vi "Konfig Dateien laden-speichern.vi"(6 "Aktion":T1=enum."laden", 8 "Fehler (Eingang)":errorcluster, 11 "Software Version":string) -> (0 "Fehler (Ausgang)":errorcluster)   [LabVIEW 2020, in "Konfig-Dateien.lvlib"]
uses:
  Konfig-Dateien.lvlib
  Aktionen Konfig.ctl
  Betriebsstundenzaehler/FGV BSZ Aktionen.ctl
  Stickstoff Befuellung/Aktionen Stockstoff Befuellung.ctl
  FGV Betriebsdaten Aktionen.ctl
  Allgemein/FGV Zustaende Aktionen.ctl
  SysLog/SysLog Interface cRIO.ctl
  Externe Stickstoff Befuellung/Aktionen Externe Stockstoff Befuellung.ctl
  CAN Interface/FGV CAN Daten Aktionen.ctl
  <vilib>/Utility/config.llb/Write Key (U32).vi
  <vilib>/Utility/config.llb/Write Key (String).vi
  Betriebsstundenzaehler/Betriebsstundenzaehler.lvlib
  Stickstoff Befuellung/Stickstoff Befuellung.lvlib
  Allgemein/Allgemein.lvlib
  SysLog/SysLog_cRIO.lvlib
  <vilib>/Utility/config.llb/NI_LVConfig.lvlib
  Externe Stickstoff Befuellung/Externe Stickstoff Befuellung.lvlib
  CAN Interface/CAN Interface.lvlib
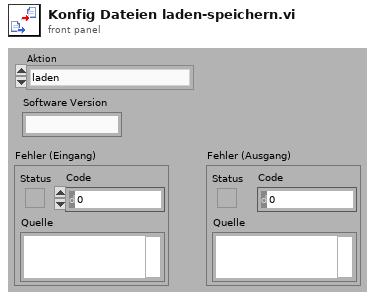
[diagram p1: front panel]
types:
  T1 = typedef "Konfig-Dateien.lvlib/Aktionen Konfig.ctl" = enum16{"lesen", "laden", "speichern  System.ini", "speichern Anlagengrenzw.", "speichern PID + Sonstige", "speichern BSZ BMP", "speichern BSZ FT-IR", "speichern Stickstoff Bef.", "speichern Ext. Stickstoff Bef.", "speichern CAN_Konfig"}
  T2 = typedef "Allgemein.lvlib/FGV Zustaende Aktionen.ctl" = enum16{"lesen", "Zustand PC", "Zustand cRIO", "Bildnummer", "Samplepoint", "Sysloglevel"}
  T3 = typedef "Konfig-Dateien.lvlib/FGV Betriebsdaten Aktionen.ctl" = enum16{"lesen", "Anlagengrenzw.", "PID Param.", "Sonstige", "Sensor Para."}
  T4 = typedef "Stickstoff Befuellung.lvlib/Aktionen Stockstoff Befuellung.ctl" = enum16{"lesen", "Befüllen vorbereiten", "Befüllen", "Befüllen beenden", "Warten", "deaktiviert", "initialisieren", "anstehender Fehler"}
  T5 = typedef "Betriebsstundenzaehler.lvlib/FGV BSZ Aktionen.ctl" = enum16{"Lesen", "Initialisieren", "Starten Pumpe", "Zählen Pumpe", "Starten FT-IR", "Zählen FT-IR"}
  T6 = typedef "CAN Interface.lvlib/FGV CAN Daten Aktionen.ctl" = enum16{"lesen", "Daten", "Konfig", "laden", "speichern", "Status"}
  T7 = typedef "Externe Stickstoff Befuellung.lvlib/Aktionen Externe Stockstoff Befuellung.ctl" = enum16{"lesen", "Befüllen vorbereiten", "Befüllen", "Befüllen beenden", "Warten", "deaktiviert", "initialisieren"}
  T8 = typedef "SysLog_cRIO.lvlib/SysLog Interface cRIO.ctl" = cluster{"FehlermeldungsCode":i32, "ErfolgsmeldungsCode":i32, "ParameterListenString":string, "intern":bool}
  T9 = typedef "Anlagengrenzwerte.lvlib/Anlagen-Grenzwerte Anzeige.ctl" = cluster{"Eingangsdruck FT-IR:":T10, "Durchfluss FT-IR:":T10, "Durchfluss CalGas:":T10, "Druck Ausgang:":T10, "Druck Kalter Block:":T10, "Heizleitungen intern:":T10, "Heizleitung zu FT-IR:":T10, "Heizung Filterblock:":T10, "Heizung Pumpe:":T10, "Heizleitung Extern SP1:":T10, "Heizleitung Extern SP2:":T10, "FT-IR Heizung Messzelle:":T10, "Schaltschranktemperatur:":T10, "Gaskühler:":T10}
  T10 = typedef "Anlagengrenzwerte.lvlib/Anlagen-Parameter Anzeige.ctl" = cluster{"Sollwert":sgl, "Warn-Min":sgl, "Warn-Max":sgl, "Abschalt-Min":sgl, "Abschalt-Max":sgl, "Regler":u16}
  T11 = typedef "Erweiterte Konfig.lvlib/PID-Parameter Anzeige.ctl" = cluster{"Heizung\nFilterblock":T12, "Heizung\nPumpe":T12, "Heizung\nHeizleitungen":T12, "Heizleitung\nExtern":T12, "Heizung\nFB-Druckregler":T12}
  T12 = typedef "Erweiterte Konfig.lvlib/PID-Parameter.ctl" = cluster{"P-Anteil":T13, "I-Anteil":T13, "D-Anteil":T13, "Regelzonengr.":T13, "max. OUT":T13}
  T13 = typedef "Zahlen-Eingabefeld.ctl" = sgl
  T14 = typedef "Erweiterte Konfig.lvlib/Sonstige Parameter.ctl" = cluster{"Lüfter langsam":sgl, "Lüfter schnell":sgl, "FT-IR Kühlung Soll":sgl, "FT-IR Kühlung Max":sgl, "Überwachung":T15, "Befüllung aktiv":T16, "Stickstoff Befüllzeit":sgl, "Befüllintervall":sgl, "Kalibrierwert FT-IR":sgl, "Offset Ausgang":sgl, "Offset FT-IR":sgl, "Offset Druck FT-IR":sgl, "Dichtheitstest Zeit":sgl, "Dichtheitstest Abfall":sgl, "Dichtheitstest Umfang":T17, "Offset Umgebung":sgl, "Max Taupunkt":sgl, "Pumpendrehzahl":sgl, "ext. Befüllung":T16, "Ext. Stickstoff Befüllzeit":sgl}
  T15 = typedef "Auswahlfeld.ctl" = u16
  T16 = typedef "LogKonfig.lvlib/Auswahlfeld aktiviert-deaktiviert.ctl" = u16
  T17 = typedef "Erweiterte Konfig.lvlib/Dichtheitstest Umfang.ctl" = u16
  T18 = cluster{"PID-Parameter Anzeige":T11, "Sonstige":T14, "Parameter Sensoren":cluster{"Kal.Durchfl.FTIR":sgl, "Kal.Durchfl.PMA":sgl, "Offset Durchfl.FTIR":sgl, "Offset Druck Ausgang":sgl, "Offset Druck Umgebung":sgl, "Offset Durchfl.PMA":sgl, "Offset Druck CG PMA":sgl, "Offset Druck CG":sgl, "Offset Druck FTIR IAG":sgl, "Druck Kalter Block":sgl}}
  T19 = typedef "Stickstoff Befuellung.lvlib/Stickstoff Befuellzeiten.ctl" = cluster{"Zeitstempel 1":timestamp, "Zeitstempel 2":timestamp, "Befülldauer":sgl}
  T20 = typedef "CAN Konfig.lvlib/Konfig Daten PC.ctl" = cluster{"Baude Rate":T21, "COM state":u8, "Frame-ID FTIR Start":u32, "Frame-ID FTIR End":u32, "Frame-ID Status Start":u32, "Frame-ID Status End":u32, "Zustand Information":u32, "Aktion":u32, "Frame-ID FTIR Arry":u32[], "Frame-ID Status Arry":u32[], "GPS Start":u32, "Interface":refnum<k21>}
  T21 = typedef "CAN Interface.lvlib/Baude Rate.ctl" = u32
  T22 = cluster{"Kal.Durchfl.FTIR":sgl, "Kal.Durchfl.PMA":sgl, "Offset Durchfl.FTIR":sgl, "Offset Druck Ausgang":sgl, "Offset Druck Umgebung":sgl, "Offset Durchfl.PMA":sgl, "Offset Druck CG PMA":sgl, "Offset Druck CG":sgl, "Offset Druck FTIR IAG":sgl, "Druck Kalter Block":sgl}
  T23 = cluster{"SysLogLevel":u16, "Software Version":string}
  T24 = cluster{"Lüfter langsam":sgl, "Lüfter schnell":sgl, "FT-IR Kühlung Soll":sgl, "FT-IR Kühlung Max":sgl, sgl, sgl, "Stickstoff Befüllzeit":sgl, "Befüllintervall":sgl, "Kalibrierwert FT-IR":sgl, "Offset Ausgang":sgl, "Offset FT-IR":sgl, "Offset Druck FT-IR":sgl, "Dichtheitstest Zeit":sgl, "Dichtheitstest Abfall":sgl, sgl, "Offset Umgebung":sgl, "Max Taupunkt":sgl, "Pumpendrehzahl":sgl, sgl, "Ext. Stickstoff Befüllzeit":sgl}
  T25 = cluster{"Sollwert":sgl, "Warn-Min":sgl, "Warn-Max":sgl, "Abschalt-Min":sgl, "Abschalt-Max":sgl, "Regler":sgl}
  T26 = typedef "NI_LVConfig.lvlib/Config Data RefNum.ctl" = refnum<k1>
  T27 = typedef "Erweiterte Konfig.lvlib/Parameter Sensoren.ctl" = cluster{"Kal.Durchfl.FTIR":sgl, "Kal.Durchfl.PMA":sgl, "Offset Durchfl.FTIR":sgl, "Offset Druck Ausgang":sgl, "Offset Druck Umgebung":sgl, "Offset Durchfl.PMA":sgl, "Offset Druck CG PMA":sgl, "Offset Druck CG":sgl, "Offset Druck FTIR IAG":sgl, "Druck Kalter Block":sgl}
  T28 = cluster{"PID-Parameter":T11, "Sonstige":T14, "Parameter Sensoren":T27}
  T29 = cluster{"Befüllen 1":timestamp, "Befüllen 2":timestamp, "Befülldauer":sgl}
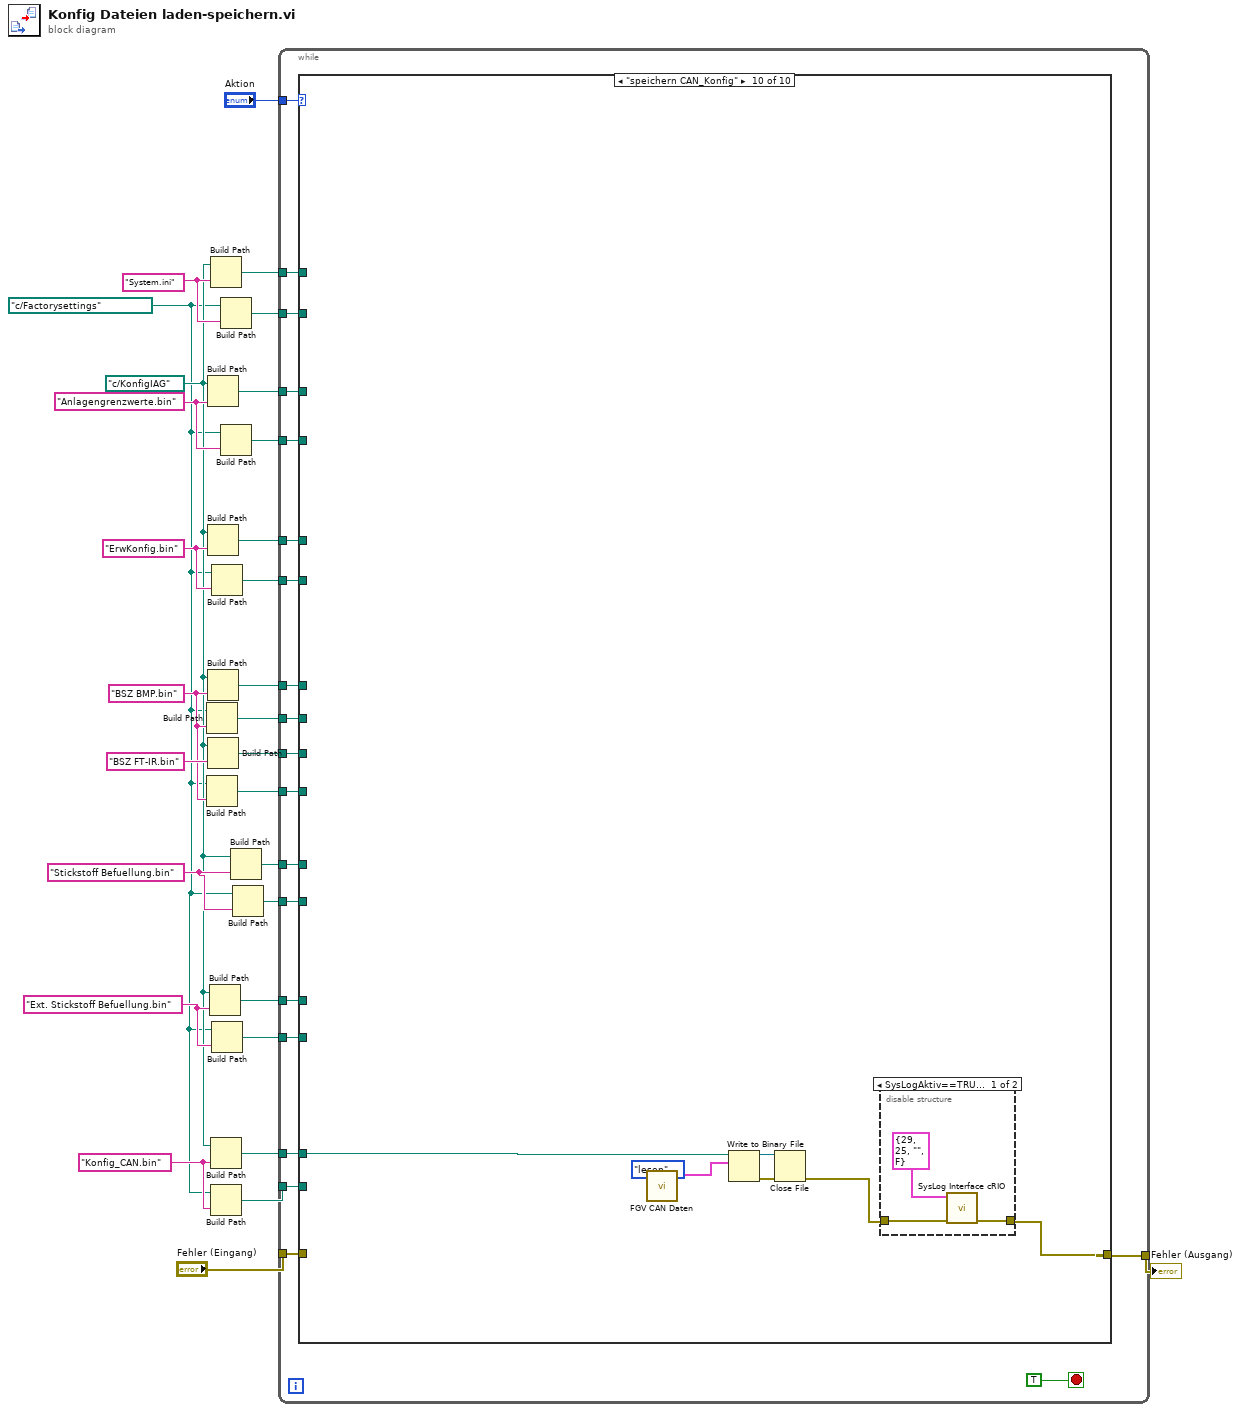
[diagram p0: block diagram]
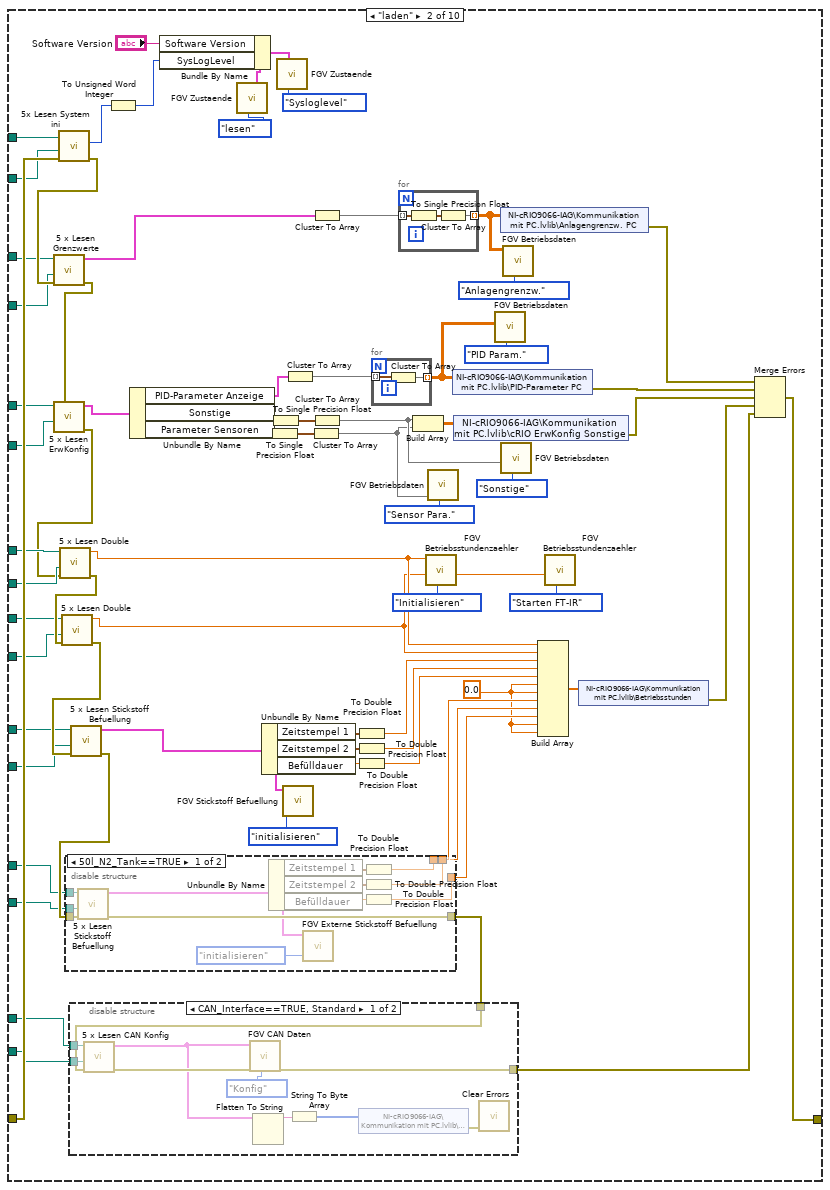
[diagram p3: hidden frame]
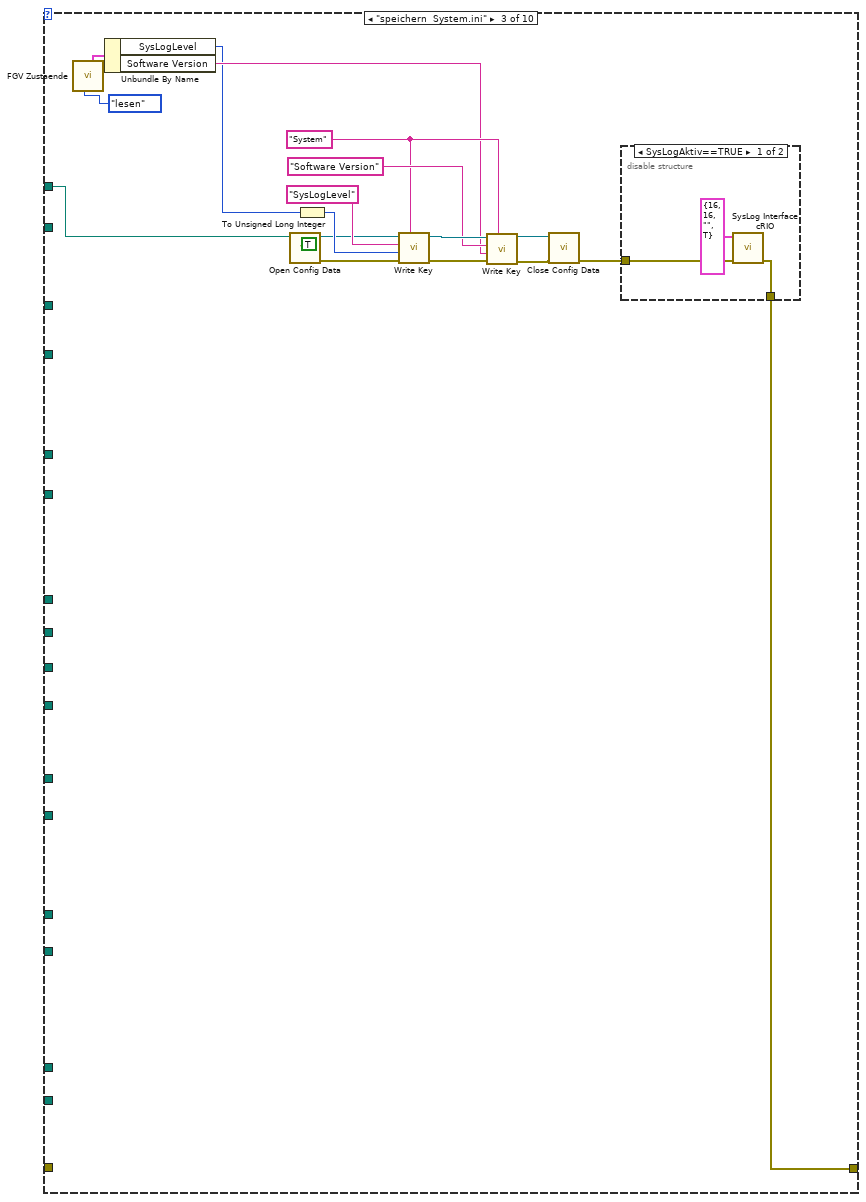
[diagram p6: hidden frame]
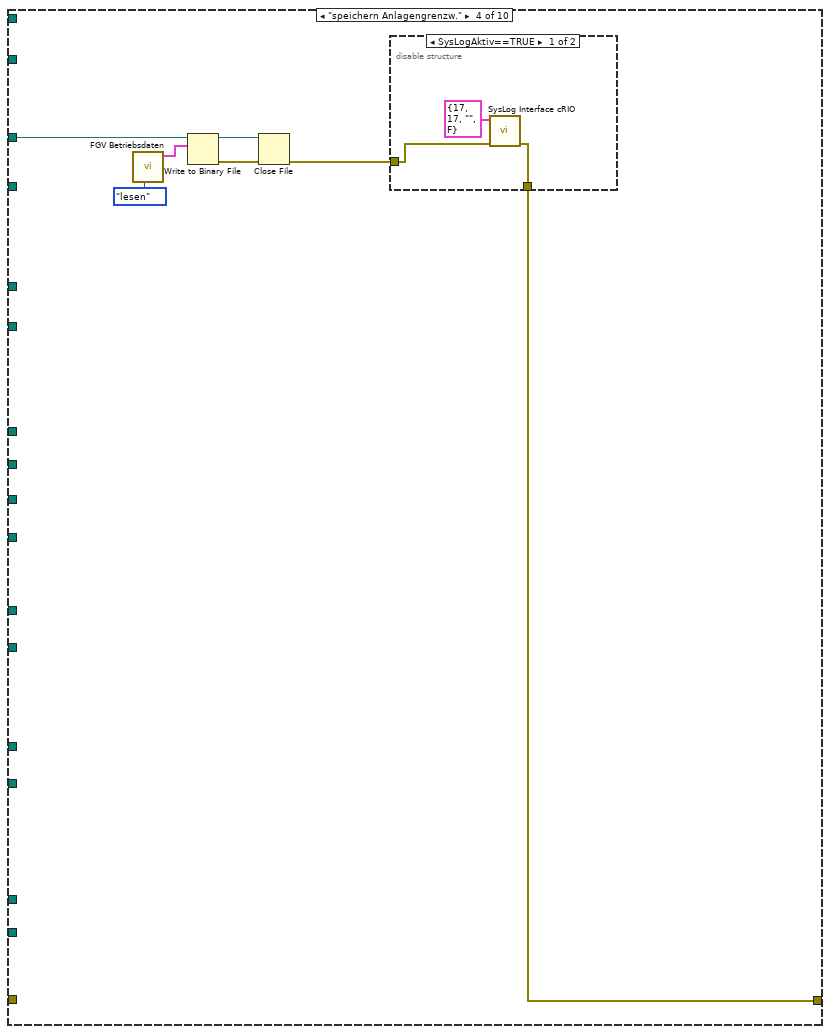
[diagram p8: hidden frame]
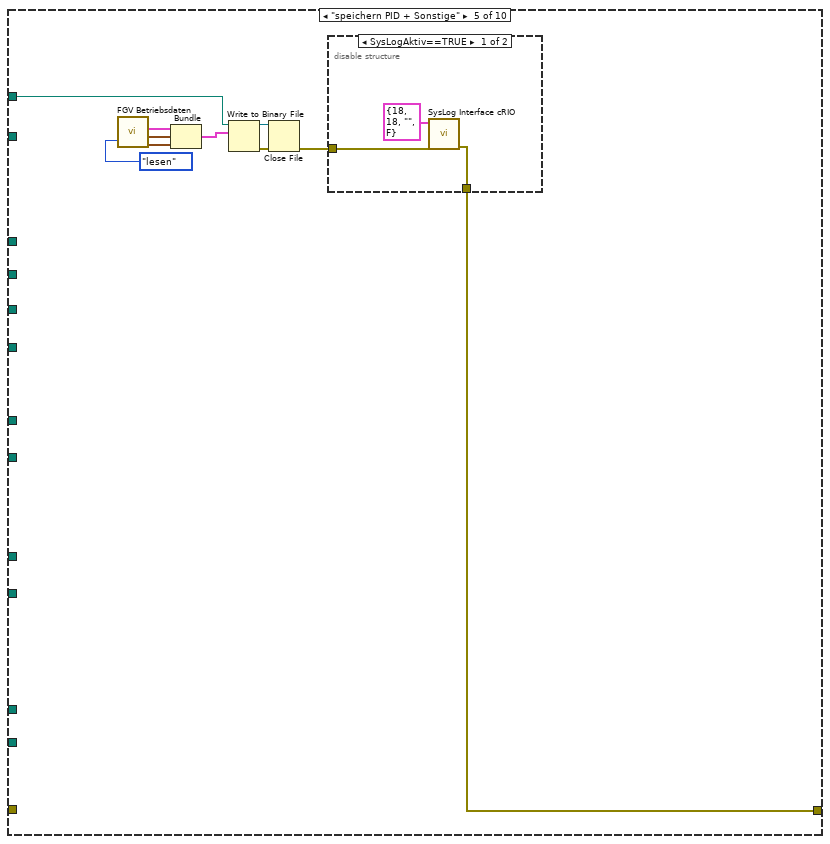
[diagram p10: hidden frame]
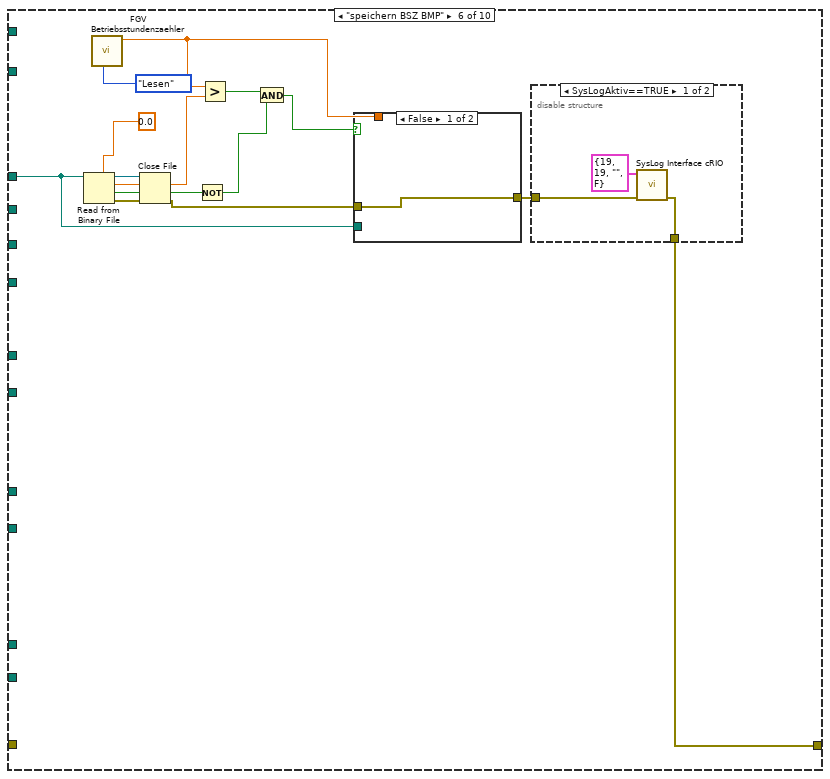
[diagram p12: hidden frame]
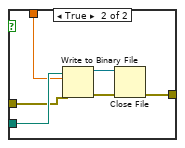
[diagram p14: hidden frame]
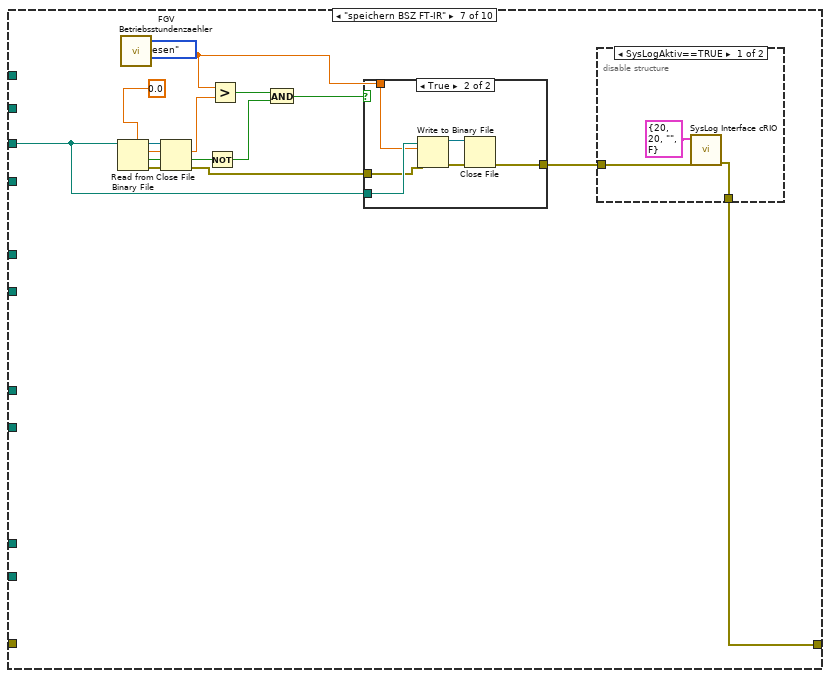
[diagram p15: hidden frame]
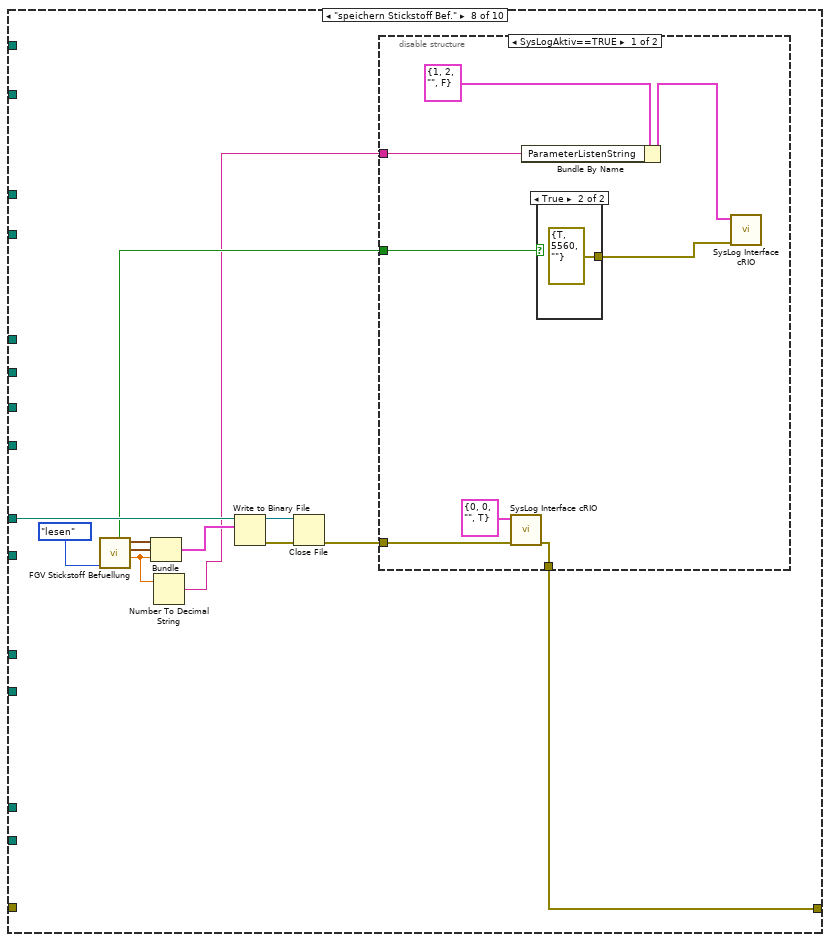
[diagram p18: hidden frame]
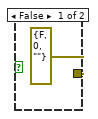
[diagram p19: hidden frame]
diagram:
  w5 = "Konfig_CAN.bin" ("Dateiname")
  w8 = "Ext. Stickstoff Befuellung.bin" ("Dateiname")
  w3 = path "c:/Factorysettings" ("Applikation:Verzeichnispfad")
  w21 = "System.ini" ("Name oder relativer Pfad")
  w13 = "Stickstoff Befuellung.bin" ("Dateiname")
  w15 = "BSZ BMP.bin" ("Dateiname")
  w16 = "ErwKonfig.bin" ("Name oder relativer Pfad")
  w4 = path "c:/KonfigIAG" ("Applikation:Verzeichnispfad")
  w19 = "Anlagengrenzwerte.bin" ("Name oder relativer Pfad")
  n1 = Build Path(base path=w3, name or relative path=w15) -> (appended path=w9:path)
  n2 = Build Path(base path=w3, name or relative path=w15) -> (appended path=w11:path)
  n3 = Build Path(base path=w4, name or relative path=w19) -> (appended path=w28:path)
  n4 = Build Path(base path=w4, name or relative path=w16) -> (appended path=w17:path)
  n5 = Build Path(base path=w4, name or relative path=w15) -> (appended path=w27:path)
  n6 = Build Path(base path=w4, name or relative path="BSZ FT-IR.bin" ("Dateiname")) -> (appended path=w25:path)
  n7 = Build Path(base path=w4, name or relative path=w8) -> (appended path=w7:path)
  n8 = Build Path(base path=w4, name or relative path=w21) -> (appended path=w24:path)
  n9 = Build Path(base path=w4, name or relative path=w5) -> (appended path=w2:path)
  n10 = Build Path(base path=w3, name or relative path=w5) -> (appended path=w1:path)
  n11 = Build Path(base path=w3, name or relative path=w16) -> (appended path=w10:path)
  n12 = Build Path(base path=w3, name or relative path=w8) -> (appended path=w6:path)
  n13 = Build Path(base path=w3, name or relative path=w21) -> (appended path=w20:path)
  n14 = Build Path(base path=w3, name or relative path=w19) -> (appended path=w18:path)
  n15 = Build Path(base path=w4, name or relative path=w13) -> (appended path=w14:path)
  n16 = Build Path(base path=w3, name or relative path=w13) -> (appended path=w12:path)
  n17 = while {
    tunnel: "Aktion" -> [w46]
    tunnel: w17 -> [w47]
    tunnel: w28 -> [w48]
    tunnel: w27 -> [w45]
    tunnel: w25 -> [w44]
    tunnel: w14 -> [w43]
    tunnel: w24 -> [w42]
    tunnel: [w41] -> w23
    tunnel: "Fehler (Eingang)" -> [w40]
    tunnel: w20 -> [w39]
    tunnel: w18 -> [w38]
    tunnel: w12 -> [w37]
    tunnel: w11 -> [w36]
    tunnel: w10 -> [w35]
    tunnel: w9 -> [w34]
    tunnel: w7 -> [w33]
    tunnel: w6 -> [w32]
    tunnel: w2 -> [w31]
    tunnel: w1 -> [w30]
    stop <- TRUE stop-if-true
    n18 = case shown="\"speichern CAN_Konfig\"" w46 {
      tunnel: w48 -> [_ w79 _ w178 _ _ _ _ _ _]
      tunnel: w47 -> [_ w76 _ _ w191 _ _ _ _ _]
      tunnel: w45 -> [_ w73 _ _ _ w204 _ _ _ _]
      tunnel: w44 -> [_ w68 _ _ _ _ w226 _ _ _]
      tunnel: w43 -> [_ w64 _ _ _ _ _ w254 _ _]
      tunnel: w42 -> [_ w92 w153 _ _ _ _ _ _ _]
      tunnel: [w50 w84 w151 w175 w185 w198 w222 w249 w275 w287] -> w41
      tunnel: w40 -> [w50 w83 _ _ _ _ _ _ _ _]
      tunnel: w39 -> [_ w78 _ _ _ _ _ _ _ _]
      tunnel: w38 -> [_ w80 _ _ _ _ _ _ _ _]
      tunnel: w37 -> [_ w63 _ _ _ _ _ _ _ _]
      tunnel: w36 -> [_ w67 _ _ _ _ _ _ _ _]
      tunnel: w35 -> [_ w75 _ _ _ _ _ _ _ _]
      tunnel: w34 -> [_ w72 _ _ _ _ _ _ _ _]
      tunnel: w33 -> [_ w60 _ _ _ _ _ _ w270 _]
      tunnel: w32 -> [_ w59 _ _ _ _ _ _ _ _]
      tunnel: w31 -> [_ w54 _ _ _ _ _ _ _ w289]
      tunnel: w30 -> [_ w53 _ _ _ _ _ _ _ _]
      frame "lesen", Default {
      }
      frame "laden" {
        w55 = 0.0 ("Element")
        n19 = call "5x Lesen System ini.vi"("Fehler (Eingang, kein Fehler)"=w83, "Factorysettings"=w78, "appended path"=w92) -> ("Fehler (Ausgang)"=w81:errorcluster, "Sys Log Level"=w91:i32)  [unwired: 6 in, 1 out]
        n20 = call "5 x Lesen Grenzwerte.vi"("Fehler (Eingang, kein Fehler)"=w81, "Factorysettings"=w80, "appended path"=w79) -> ("Fehler (Ausgang)"=w77:errorcluster, "Anlagen-Grenzwerte Anzeige"=w82:T9)  [unwired: 6 in, 1 out]
        n21 = call "5 x Lesen ErwKonfig.vi"("Fehler (Eingang, kein Fehler)"=w77, "Factorysettings"=w75, "appended path"=w76) -> ("Fehler (Ausgang)"=w71:errorcluster, "Erw. Konfig"=w74:T18)  [unwired: 6 in, 1 out]
        n22 = call "5 x Lesen Double.vi"("Fehler (Eingang, kein Fehler)"=w71, "Factorysettings"=w72, "appended path"=w73) -> ("Fehler (Ausgang)"=w69:errorcluster, "Double (Ausgang)"=w70:dbl)  [unwired: 6 in, 1 out]
        n23 = call "5 x Lesen Double.vi"("Fehler (Eingang, kein Fehler)"=w69, "Factorysettings"=w67, "appended path"=w68) -> ("Fehler (Ausgang)"=w65:errorcluster, "Double (Ausgang)"=w66:dbl)  [unwired: 6 in, 1 out]
        n24 = call "5 x Lesen Stickstoff Befuellung.vi"("Fehler (Eingang, kein Fehler)"=w65, "Factorysettings"=w63, "appended path"=w64) -> ("Fehler (Ausgang)"=w61:errorcluster, "Stiskstoff Befüllzeiten"=w62:T19)  [unwired: 6 in, 1 out]
        n25 = disable-structure shown="50l_N2_Tank==TRUE" {
          disable-tunnel: w61 -> [w142 _]
          disable-tunnel: [w141 _] -> w52
          disable-tunnel: w60 -> [w138 _]
          disable-tunnel: w59 -> [w137 _]
          disable-tunnel: [w136 _] -> w58
          disable-tunnel: [w135 _] -> w57
          disable-tunnel: [w134 _] -> w56
          frame condition #0 {
            n26 = call "5 x Lesen Stickstoff Befuellung.vi"("Fehler (Eingang, kein Fehler)"=w142, "Factorysettings"=w137, "appended path"=w138) -> ("Fehler (Ausgang)"=w141:errorcluster, "Stiskstoff Befüllzeiten"=w140:T19)  [unwired: 6 in, 1 out]
            n27 = Unbundle By Name(w140) -> ("Zeitstempel 1"=w143:timestamp, "Zeitstempel 2"=w144:timestamp, "Befülldauer"=w145:sgl)
            n28 = call "FGV Externe Stickstoff Befuellung.vi"("Aktion"=Aktionen_Externe_Stockstoff_Befuellung."initialisieren", "Stiskstoff Befüllzeiten"=w140) -> ()  [unwired: 3 in, 7 out]
            n29 = To Double Precision Float(number=w143) -> (double precision float=w136:dbl)
            n30 = To Double Precision Float(number=w144) -> (double precision float=w135:dbl)
            n31 = To Double Precision Float(number=w145) -> (double precision float=w134:dbl)
          }
          frame condition #1 (active) {
          }
        }
        n32 = disable-structure shown="CAN_Interface==TRUE, Standard" {
          disable-tunnel: w54 -> [w131 _]
          disable-tunnel: w53 -> [w130 _]
          disable-tunnel: w52 -> [w129 w133]
          disable-tunnel: [w128 w133] -> w51
          frame condition #0 {
            n33 = call "5 x Lesen CAN Konfig.vi"("Fehler (Eingang, kein Fehler)"=w129, "Factorysettings"=w130, "appended path"=w131) -> ("Fehler (Ausgang)"=w128:errorcluster, "Konfig Daten 2"=w126:T20)  [unwired: 6 in, 1 out]
            n34 = call "FGV CAN Daten.vi"("Aktionen"=FGV_CAN_Daten_Aktionen."Konfig", "Konfig Daten 2"=w126) -> ()  [unwired: 7 in, 3 out]
            n35 = Flatten To String(anything=w126) -> (data string=w127:string)  [unwired: 3 in, 2 out]
            n36 = String To Byte Array(string=w127) -> (unsigned byte array=w125:u8[])
            n37 = shared-variable "NI-cRIO9066-IAG\\Kommunikation mit PC.lvlib\\CAN_Konfig"(w125) -> (error out=w124:errorcluster)  [unwired: 1 in]
            n38 = call <vilib>:"Clear Errors.vi"("error in (no error)"=w124) -> ()  [unwired: 5 in, 2 out]
          }
          frame condition #1 (active) {
          }
        }
        n39 = To Unsigned Word Integer(number=w91) -> (unsigned 16bit integer=w85:u16)
        n40 = Unbundle By Name(w74) -> ("PID-Parameter Anzeige"=w110:T11, "Sonstige"=w108:T14, "Parameter Sensoren"=w97:T22)
        n41 = call "FGV Zustaende.vi"("Aktionen"=FGV_Zustaende_Aktionen."lesen") -> ("SL SV Cluster"=w88:T23)  [unwired: 6 in, 4 out]
        n42 = Bundle By Name(cluster=w88, "Software Version"="Software Version", "SysLogLevel"=w85) -> (w86:T23)
        n43 = Unbundle By Name(w62) -> ("Zeitstempel 1"=w118:timestamp, "Zeitstempel 2"=w117:timestamp, "Befülldauer"=w116:sgl)
        n44 = To Single Precision Float(number=w97) -> (single precision float=w98:T22)
        n45 = To Single Precision Float(number=w108) -> (single precision float=w109:T24)
        n46 = call "FGV Zustaende.vi"("Aktionen"=FGV_Zustaende_Aktionen."Sysloglevel", "SL SV Cluster"=w86) -> ()  [unwired: 5 in, 5 out]
        n47 = call "FGV Stickstoff Befuellung.vi"("Aktion"=Aktionen_Stockstoff_Befuellung."initialisieren", "Stiskstoff Befüllzeiten"=w62) -> ()  [unwired: 3 in, 7 out]
        n48 = Cluster To Array(cluster=w110) -> (array=w111:T12[])
        n49 = Cluster To Array(cluster=w98) -> (array=w93:sgl[])
        n50 = Cluster To Array(cluster=w82) -> (array=w112:T10[])
        n51 = Cluster To Array(cluster=w109) -> (array=w96:sgl[])
        n52 = To Double Precision Float(number=w118) -> (double precision float=w115:dbl)
        n53 = To Double Precision Float(number=w117) -> (double precision float=w114:dbl)
        n54 = To Double Precision Float(number=w116) -> (double precision float=w113:dbl)
        n55 = for {
          tunnel: w111 -> [w147] mode=indexing
          tunnel: [w146] -> w103 mode=indexing
          n56 = Cluster To Array(cluster=w147) -> (array=w146:T13[])
        }
        n57 = for {
          tunnel: w112 -> [w150] mode=indexing
          tunnel: [w148] -> w106 mode=indexing
          n58 = To Single Precision Float(number=w150) -> (single precision float=w149:T25)
          n59 = Cluster To Array(cluster=w149) -> (array=w148:sgl[])
        }
        n60 = Build Array(w96, w93) -> (w94:sgl[][])
        n61 = call "FGV Betriebsstundenzaehler.vi"("BSZ Aktionen"=FGV_BSZ_Aktionen."Initialisieren", "Betriebsstunden FT-IR"=w66, "Betriebsstunden Pumpe"=w70) -> ("Betriebsstunden FT-IR"=w121:dbl)  [unwired: 7 in, 1 out]
        n62 = call "FGV Betriebsdaten.vi"("Aktionen"=FGV_Betriebsdaten_Aktionen."Sensor Para.", "Parameter Sensoren"=w93) -> ()  [unwired: 6 in, 4 out]
        n63 = shared-variable "NI-cRIO9066-IAG\\Kommunikation mit PC.lvlib\\PID-Parameter PC"(w103) -> (error out=w100:errorcluster)  [unwired: 1 in]
        n64 = shared-variable "NI-cRIO9066-IAG\\Kommunikation mit PC.lvlib\\cRIO ErwKonfig Sonstige"(w94) -> (error out=w101:errorcluster)  [unwired: 1 in]
        n65 = call "FGV Betriebsdaten.vi"("Aktionen"=FGV_Betriebsdaten_Aktionen."PID Param.", "PID-Parameter"=w103) -> ()  [unwired: 6 in, 4 out]
        n66 = shared-variable "NI-cRIO9066-IAG\\Kommunikation mit PC.lvlib\\Anlagengrenzw. PC"(w106) -> (error out=w99:errorcluster)  [unwired: 1 in]
        n67 = call "FGV Betriebsdaten.vi"("Aktionen"=FGV_Betriebsdaten_Aktionen."Sonstige", "Sonstige"=w96) -> ()  [unwired: 6 in, 4 out]
        n68 = call "FGV Betriebsdaten.vi"("Aktionen"=FGV_Betriebsdaten_Aktionen."Anlagengrenzw.", "Anlagen-Grenzwerte"=w106) -> ()  [unwired: 6 in, 4 out]
        n69 = Build Array(w70, w66, w115, w114, w113, w55, w55, w58, w57, w56, w55, w55) -> (w120:dbl[])
        n70 = call "FGV Betriebsstundenzaehler.vi"("BSZ Aktionen"=FGV_BSZ_Aktionen."Starten FT-IR", "Betriebsstunden FT-IR"=w121) -> ()  [unwired: 8 in, 2 out]
        n71 = shared-variable "NI-cRIO9066-IAG\\Kommunikation mit PC.lvlib\\Betriebsstunden"(w120) -> (error out=w102:errorcluster)  [unwired: 1 in]
        n72 = Merge Errors(w99, w100, w101, w102, w51) -> (w84:errorcluster)
      }
      frame "speichern  System.ini" {
        w163 = "System" ("section")
        n73 = call "FGV Zustaende.vi"("Aktionen"=FGV_Zustaende_Aktionen."lesen") -> ("SL SV Cluster"=w156:T23)  [unwired: 6 in, 4 out]
        n74 = Unbundle By Name(w156) -> ("SysLogLevel"=w154:u16, "Software Version"=w155:string)
        n75 = call <vilib>:"Open Config Data.vi"("create file if necessary (T)"=TRUE, "configuration file path"=w153) -> ("error out"=w158:errorcluster, "refnum"=w157:T26)  [unwired: 7 in, 1 out]
        n76 = To Unsigned Long Integer(number=w154) -> (unsigned 32bit integer=w160:u32)
        n77 = call-poly <vilib>:"Write Key.vi"("section"=w163, "error in (no error)"=w158, "value"=w160, "key"="SysLogLevel", "refnum"=w157) -> ("error out"=w161:errorcluster, "refnum out"=w165:T26)  [unwired: 4 in, 1 out]
        n78 = call-poly <vilib>:"Write Key.vi"("section"=w163, "error in (no error)"=w161, "value"=w155, "key"="Software Version", "refnum"=w165) -> ("error out"=w162:errorcluster, "refnum out"=w166:T26)  [unwired: 4 in, 1 out]
        n79 = call <vilib>:"Close Config Data.vi"("error in (no error)"=w162, "refnum"=w166) -> ("error out"=w152:errorcluster)  [unwired: 8 in, 1 out]
        n80 = disable-structure shown="SysLogAktiv==TRUE" {
          disable-tunnel: w152 -> [w171 _]
          disable-tunnel: [w170 _] -> w151
          frame condition #0 (active) {
            n81 = call "SysLog Interface cRIO.vi"("Fehler (in)"=w171, "Cluster (in)"=T8 {"FehlermeldungsCode"=16, "ErfolgsmeldungsCode"=16, "ParameterListenString"="", "intern"=TRUE}) -> ("Fehler (Ausgang)"=w170:errorcluster)  [unwired: 9 in]
          }
          frame condition #1 {
          }
        }
      }
      frame "speichern Anlagengrenzw." {
        n82 = call "FGV Betriebsdaten.vi"("Aktionen"=FGV_Betriebsdaten_Aktionen."lesen") -> ("Anlagen-Grenzwerte"=w176:T9)  [unwired: 7 in, 3 out]
        n83 = Write to Binary File(file (use dialog)=w178, data=w176) -> (refnum out=w174:refnum<file>, error out=w173:errorcluster)  [unwired: 1 in, 4 out]
        n84 = Close File(refnum=w174, error in=w173) -> (error out=w172:errorcluster)  [unwired: 1 out]
        n85 = disable-structure shown="SysLogAktiv==TRUE" {
          disable-tunnel: w172 -> [w181 _]
          disable-tunnel: [w180 _] -> w175
          frame condition #0 (active) {
            n86 = call "SysLog Interface cRIO.vi"("Fehler (in)"=w181, "Cluster (in)"=T8 {"FehlermeldungsCode"=17, "ErfolgsmeldungsCode"=17, "ParameterListenString"="", "intern"=FALSE}) -> ("Fehler (Ausgang)"=w180:errorcluster)  [unwired: 9 in]
          }
          frame condition #1 {
          }
        }
      }
      frame "speichern PID + Sonstige" {
        n87 = call "FGV Betriebsdaten.vi"("Aktionen"=FGV_Betriebsdaten_Aktionen."lesen") -> ("Parameter Sensoren"=w186:T27, "Sonstige"=w188:T14, "PID-Parameter"=w189:T11)  [unwired: 7 in, 1 out]
        n88 = Bundle("PID-Parameter"=w189, "Sonstige"=w188, "Parameter Sensoren"=w186) -> (w187:T28)  [unwired: 1 in]
        n89 = Write to Binary File(file (use dialog)=w191, data=w187) -> (refnum out=w184:refnum<file>, error out=w183:errorcluster)  [unwired: 1 in, 4 out]
        n90 = Close File(refnum=w184, error in=w183) -> (error out=w182:errorcluster)  [unwired: 1 out]
        n91 = disable-structure shown="SysLogAktiv==TRUE" {
          disable-tunnel: w182 -> [w194 _]
          disable-tunnel: [w193 _] -> w185
          frame condition #0 (active) {
            n92 = call "SysLog Interface cRIO.vi"("Fehler (in)"=w194, "Cluster (in)"=T8 {"FehlermeldungsCode"=18, "ErfolgsmeldungsCode"=18, "ParameterListenString"="", "intern"=FALSE}) -> ("Fehler (Ausgang)"=w193:errorcluster)  [unwired: 9 in]
          }
          frame condition #1 {
          }
        }
      }
      frame "speichern BSZ BMP" {
        n93 = Read from Binary File(5:0.0 ("Betriebsstunden FT-IR"), 11:w204) -> (0:w196:errorcluster, 1:w206:bool, 2:w202:dbl, 3:w197:refnum<file>)  [unwired: 4 in]
        n94 = call "FGV Betriebsstundenzaehler.vi"("BSZ Aktionen"=FGV_BSZ_Aktionen."Lesen") -> ("Betriebsstunden Pumpe"=w201:dbl)  [unwired: 9 in, 1 out]
        n95 = Close File(refnum=w197, error in=w196) -> (error out=w195:errorcluster)  [unwired: 1 out]
        n96 = Not(x=w206) -> (.not. x?=w203:bool)
        n97 = Greater?(x=w201, y=w202) -> (0:w207:bool)
        n98 = And(x=w207, y=w203) -> (x .and. y?=w200:bool)
        n99 = case shown="False" w200 {
          tunnel: w204 -> [_ w218]
          tunnel: w201 -> [_ w217]
          tunnel: w195 -> [w212 w216]
          tunnel: [w212 w213] -> w199
          frame False {
          }
          frame True {
            n100 = Write to Binary File(file (use dialog)=w218, data=w217, error in=w216) -> (refnum out=w215:refnum<file>, error out=w214:errorcluster)  [unwired: 4 out]
            n101 = Close File(refnum=w215, error in=w214) -> (error out=w213:errorcluster)  [unwired: 1 out]
          }
        }
        n102 = disable-structure shown="SysLogAktiv==TRUE" {
          disable-tunnel: w199 -> [w211 _]
          disable-tunnel: [w210 _] -> w198
          frame condition #0 (active) {
            n103 = call "SysLog Interface cRIO.vi"("Fehler (in)"=w211, "Cluster (in)"=T8 {"FehlermeldungsCode"=19, "ErfolgsmeldungsCode"=19, "ParameterListenString"="", "intern"=FALSE}) -> ("Fehler (Ausgang)"=w210:errorcluster)  [unwired: 9 in]
          }
          frame condition #1 {
          }
        }
      }
      frame "speichern BSZ FT-IR" {
        n104 = Read from Binary File(5:0.0 ("Betriebsstunden FT-IR"), 11:w226) -> (0:w221:errorcluster, 1:w229:bool, 2:w228:dbl, 3:w220:refnum<file>)  [unwired: 4 in]
        n105 = call "FGV Betriebsstundenzaehler.vi"("BSZ Aktionen"=FGV_BSZ_Aktionen."Lesen") -> ("Betriebsstunden FT-IR"=w225:dbl)  [unwired: 9 in, 1 out]
        n106 = Close File(refnum=w220, error in=w221) -> (error out=w219:errorcluster)  [unwired: 1 out]
        n107 = Not(x=w229) -> (.not. x?=w230:bool)
        n108 = Greater?(x=w225, y=w228) -> (0:w231:bool)
        n109 = And(x=w231, y=w230) -> (x .and. y?=w224:bool)
        n110 = case shown="True" w224 {
          tunnel: w226 -> [_ w242]
          tunnel: w225 -> [_ w241]
          tunnel: w219 -> [w236 w240]
          tunnel: [w236 w237] -> w223
          frame False {
          }
          frame True {
            n111 = Write to Binary File(file (use dialog)=w242, data=w241, error in=w240) -> (refnum out=w239:refnum<file>, error out=w238:errorcluster)  [unwired: 4 out]
            n112 = Close File(refnum=w239, error in=w238) -> (error out=w237:errorcluster)  [unwired: 1 out]
          }
        }
        n113 = disable-structure shown="SysLogAktiv==TRUE" {
          disable-tunnel: w223 -> [w235 _]
          disable-tunnel: [w234 _] -> w222
          frame condition #0 (active) {
            n114 = call "SysLog Interface cRIO.vi"("Fehler (in)"=w235, "Cluster (in)"=T8 {"FehlermeldungsCode"=20, "ErfolgsmeldungsCode"=20, "ParameterListenString"="", "intern"=FALSE}) -> ("Fehler (Ausgang)"=w234:errorcluster)  [unwired: 9 in]
          }
          frame condition #1 {
          }
        }
      }
      frame "speichern Stickstoff Bef." {
        n115 = call "FGV Stickstoff Befuellung.vi"("Aktion"=Aktionen_Stockstoff_Befuellung."lesen") -> ("Befülldauer"=w247:sgl, "Befüllen 2"=w251:timestamp, "Befüllen 1"=w252:timestamp, "Timeout"=w248:bool)  [unwired: 4 in, 3 out]
        n116 = Bundle("Befüllen 1"=w252, "Befüllen 2"=w251, "Befülldauer"=w247) -> (w250:T29)  [unwired: 1 in]
        n117 = Number To Decimal String(number=w247) -> (decimal integer string=w246:string)  [unwired: 1 in]
        n118 = Write to Binary File(file (use dialog)=w254, data=w250) -> (refnum out=w244:refnum<file>, error out=w245:errorcluster)  [unwired: 1 in, 4 out]
        n119 = Close File(refnum=w244, error in=w245) -> (error out=w243:errorcluster)  [unwired: 1 out]
        n120 = disable-structure shown="SysLogAktiv==TRUE" {
          disable-tunnel: w243 -> [w259 _]
          disable-tunnel: [w262 _] -> w249
          disable-tunnel: w248 -> [w260 _]
          disable-tunnel: w246 -> [w256 _]
          frame condition #0 (active) {
            n121 = call "SysLog Interface cRIO.vi"("Fehler (in)"=w259, "Cluster (in)"=T8 {"FehlermeldungsCode"=0, "ErfolgsmeldungsCode"=0, "ParameterListenString"="", "intern"=TRUE}) -> ("Fehler (Ausgang)"=w262:errorcluster)  [unwired: 9 in]
            n122 = Bundle By Name(cluster=T8 {"FehlermeldungsCode"=1, "ErfolgsmeldungsCode"=2, "ParameterListenString"="", "intern"=FALSE} ("Cluster (in)"), "ParameterListenString"=w256) -> (w257:T8)
            n123 = case shown="True" w260 {
              tunnel: [errorcluster {"status"=FALSE, "code"=0, "source"=""} ("Fehlerkonstante") errorcluster {"status"=TRUE, "code"=5560, "source"=""} ("Fehlerkonstante")] -> w261
              frame False {
              }
              frame True {
              }
            }
            n124 = call "SysLog Interface cRIO.vi"("Fehler (in)"=w261, "Cluster (in)"=w257) -> ()  [unwired: 9 in, 1 out]
          }
          frame condition #1 {
          }
        }
      }
      frame "speichern Ext. Stickstoff Bef." {
        n125 = call "FGV Externe Stickstoff Befuellung.vi"("Aktion"=Aktionen_Externe_Stockstoff_Befuellung."lesen") -> ("Befülldauer"=w267:sgl, "Befüllen 2"=w268:timestamp, "Befüllen 1"=w269:timestamp, "Timeout"=w265:bool)  [unwired: 4 in, 3 out]
        n126 = Bundle("Befüllen 1"=w269, "Befüllen 2"=w268, "Befülldauer"=w267) -> (w276:T29)  [unwired: 1 in]
        n127 = Number To Decimal String(number=w267) -> (decimal integer string=w274:string)  [unwired: 1 in]
        n128 = Write to Binary File(file (use dialog)=w270, data=w276) -> (refnum out=w272:refnum<file>, error out=w273:errorcluster)  [unwired: 1 in, 4 out]
        n129 = Close File(refnum=w272, error in=w273) -> (error out=w271:errorcluster)  [unwired: 1 out]
        n130 = disable-structure shown="SysLogAktiv==TRUE" {
          disable-tunnel: w271 -> [w281 _]
          disable-tunnel: [w284 _] -> w275
          disable-tunnel: w265 -> [w282 _]
          disable-tunnel: w274 -> [w278 _]
          frame condition #0 (active) {
            n131 = call "SysLog Interface cRIO.vi"("Fehler (in)"=w281, "Cluster (in)"=T8 {"FehlermeldungsCode"=0, "ErfolgsmeldungsCode"=0, "ParameterListenString"="", "intern"=TRUE}) -> ("Fehler (Ausgang)"=w284:errorcluster)  [unwired: 9 in]
            n132 = Bundle By Name(cluster=T8 {"FehlermeldungsCode"=1, "ErfolgsmeldungsCode"=2, "ParameterListenString"="", "intern"=FALSE} ("Cluster (in)"), "ParameterListenString"=w278) -> (w279:T8)
            n133 = case shown="True" w282 {
              tunnel: [errorcluster {"status"=FALSE, "code"=0, "source"=""} ("Fehlerkonstante") errorcluster {"status"=TRUE, "code"=5560, "source"=""} ("Fehlerkonstante")] -> w283
              frame False {
              }
              frame True {
              }
            }
            n134 = call "SysLog Interface cRIO.vi"("Fehler (in)"=w283, "Cluster (in)"=w279) -> ()  [unwired: 9 in, 1 out]
          }
          frame condition #1 {
          }
        }
      }
      frame "speichern CAN_Konfig" {
        n135 = call "FGV CAN Daten.vi"("Aktionen"=FGV_CAN_Daten_Aktionen."lesen") -> ("Konfig Daten"=w290:T20)  [unwired: 8 in, 2 out]
        n136 = Write to Binary File(file (use dialog)=w289, data=w290) -> (refnum out=w291:refnum<file>, error out=w292:errorcluster)  [unwired: 1 in, 4 out]
        n137 = Close File(refnum=w291, error in=w292) -> (error out=w288:errorcluster)  [unwired: 1 out]
        n138 = disable-structure shown="SysLogAktiv==TRUE, Standard" {
          disable-tunnel: w288 -> [w296 w297]
          disable-tunnel: [w294 w297] -> w287
          frame condition #0 (active) {
            n139 = call "SysLog Interface cRIO.vi"("Fehler (in)"=w296, "Cluster (in)"=T8 {"FehlermeldungsCode"=29, "ErfolgsmeldungsCode"=25, "ParameterListenString"="", "intern"=FALSE}) -> ("Fehler (Ausgang)"=w294:errorcluster)  [unwired: 9 in]
          }
          frame condition #1 {
          }
        }
      }
    }
  }
  "Fehler (Ausgang)" <- w23
